vi "update center voltage.vi"(7 "CursLoc":cluster{"X":dbl, "Y":dbl}, 8 "错误输入（无错误）":errorcluster, 11 "Value in":T1 {"Zoom (V)" scale=0.0..1.0; "X Pos." scale=-2.0..2.0; "Y Pos." scale=-2.0..2.0}) -> (0 "错误输出":errorcluster, 3 "Value out":T1 {"Zoom (V)" scale=0.0..1.0; "X Pos." scale=-2.0..2.0; "Y Pos." scale=-2.0..2.0})   [LabVIEW 2013]
uses:
  init & communication/Setting-User input.ctl
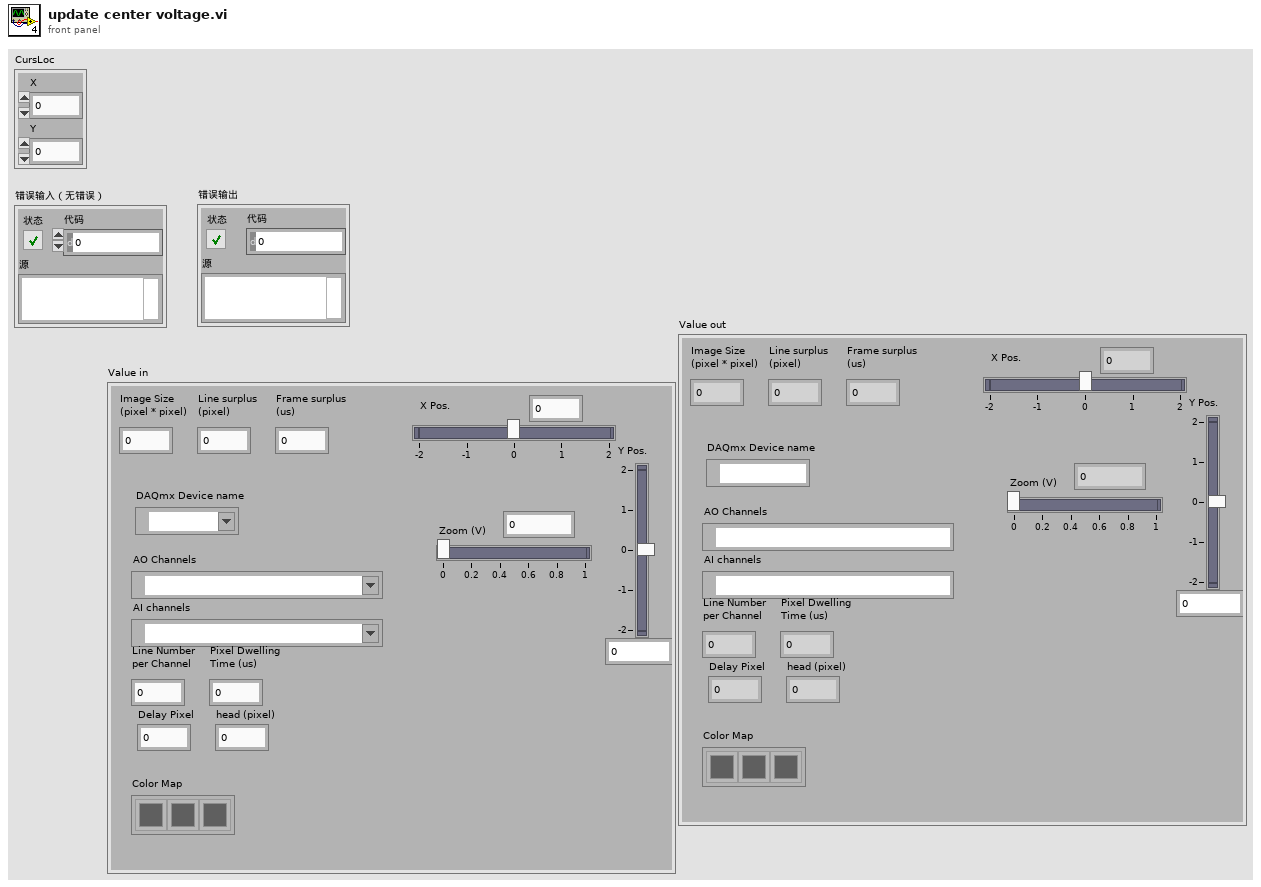
[diagram p1: front panel]
types:
  T1 = typedef "Setting-User input.ctl" = cluster{"Image Size\n(pixel * pixel)":i32, "AO Channels":tag, "Y Pos.":dbl, "X Pos.":dbl, "Line surplus\n(pixel)":i32, "Frame surplus\n(us)":i32, "AI channels":tag, "Line Number\nper Channel":i32, "Delay Pixel":i32, "Pixel Dwelling\nTime (us)":i32, "Color Map":u32[], "head (pixel)":i32, "Zoom (V)":dbl, "DAQmx Device name":tag}
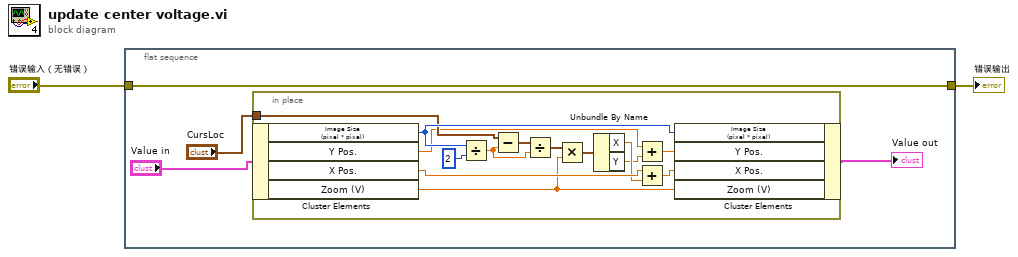
[diagram p0: block diagram]
diagram:
  n1 = flat-sequence {
    tunnel: "错误输入（无错误）" -> [w3]
    tunnel: [w3] -> w2
    frame #0 {
      n2 = in-place {
        in-place-border: "CursLoc" -> [w18]
        n3 = in-place-cluster #1("Value in") -> ("Image Size\n(pixel * pixel)"=w20:i32, "Y Pos."=w17:dbl, "X Pos."=w14:dbl, "Zoom (V)"=w10:dbl)
        n4 = Divide(x=w20, y=2) -> (x/y=w12:dbl)
        n5 = Subtract(x=w18, y=w12) -> (x-y=w13:cluster{"X":dbl, "Y":dbl})
        n6 = Divide(x=w13, y=w12) -> (x/y=w11:cluster{"X":dbl, "Y":dbl})
        n7 = Multiply(x=w11, y=w10) -> (x*y=w9:cluster{"X":dbl, "Y":dbl})
        n8 = Unbundle By Name(w9) -> ("X"=w8:dbl, "Y"=w7:dbl)
        n9 = Add(x=w17, y=w7) -> (x+y=w16:dbl)
        n10 = Add(x=w14, y=w8) -> (x+y=w15:dbl)
        n11 = in-place-cluster #1("Image Size\n(pixel * pixel)"=w20, "Y Pos."=w16, "X Pos."=w15, "Zoom (V)"=w10) -> (→"Value out":T1)
      }
    }
  }
  "错误输出" <- w2
